vi "LVClass_DataClient ctor.vi"(0 "DataClient (const)":refnum<class "DataClient.lvclass">, 5 "IP":string, 7 "port":u16, 9 "timeout":u32, 11 "error in (no error)":errorcluster) -> (4 "DataClient (new)":refnum<class "DataClient.lvclass">, 15 "error out":errorcluster)   [LabVIEW 2020, in "DataClient.lvclass"]
doc: "Client constructor from server ip adress and server port.\n\n<B>clientIn</B> : Constant Client object.\n<B>clientOut</B> : Constant Client object.\n<B>ip</B> : Server ip adress.\n<B>port</B> : Server port.\n<B>time_out</B> : Timeout (ms)."
uses:
  DataClient.lvclass
  Handle creation.ctl
  DataClient.lvclass/DataClient.ctl
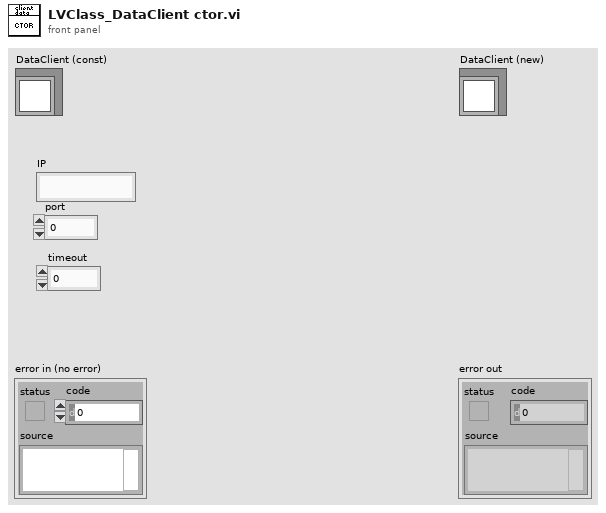
[diagram p1: front panel]
types:
  T1 = typedef "Handle creation.ctl" = enum16{"By ctor", "By write function"}
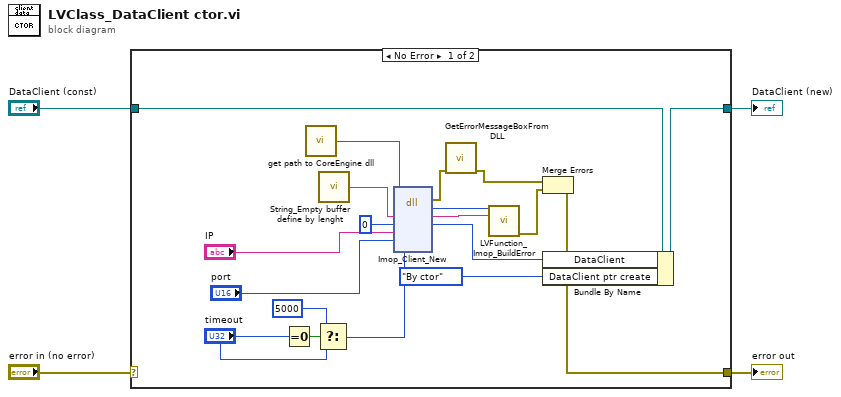
[diagram p0: block diagram]
diagram:
  n1 = case shown="No Error" "error in (no error)" {
    selector: "error in (no error)" -> [_ w25]
    tunnel: [w5 w25] -> w3
    tunnel: [w12 w24] -> w1
    tunnel: "DataClient (const)" -> [w13 w24]
    frame No Error {
      n2 = Equal To 0?(x="timeout") -> (x = 0?=w9:bool)
      n3 = call "get path to CoreEngine dll.vi"() -> ("path to wavekit library"=w18:path)  [unwired: 14 in, 1 out]
      n4 = Select(t=u32 5000, s=w9, f="timeout") -> (s? t:f=w8:u32)
      n5 = call "String_Empty buffer define by lenght.vi"() -> ("Empty buffer"=w21:string)  [unwired: 1 in]
      n6 = dll-call lib="D:/soft/HASO_v3/SVN_trunk/ImOpCoreEngine4_LV2011/DLLs/c_interface_vc100.dll" fn="Imop_Client_New"(path in=w18, "message"=w21, "Slopes Client"=0 ("Image compat"), "IP"="IP", "port"="port", "timeout"=w8) -> (error out=w17:errorcluster, "return type"=w22:i32, "message"=w23:string, "Slopes Client"=w20:i64)  [unwired: 5 in, 1 out]
      n7 = call "GetErrorMessageBoxFromDLL.vi"("error IN"=w17) -> ("error OUT"=w15:errorcluster)  [unwired: 10 in]
      n8 = call "LVFunction_Imop_BuildError.vi"("code"=w22, "String to Prepend to source (\"\")"=w23) -> ("error out"=w14:errorcluster)  [unwired: 13 in]
      n9 = Merge Errors(w15, w14) -> (w5:errorcluster)
      n10 = Bundle By Name(cluster=w13, "DataClient"=w20, "DataClient ptr create"=Handle_creation."By ctor" ("Image Compat ptr create")) -> (w12:refnum<class "DataClient.lvclass">)
    }
    frame Error {
    }
  }
  "error out" <- w3
  "DataClient (new)" <- w1
